vi "ObtainStopEvent.vi"() -> (3 "StopEvent":refnum<user-event>)   [LabVIEW 2014]
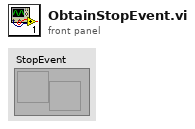
[diagram p1: front panel]
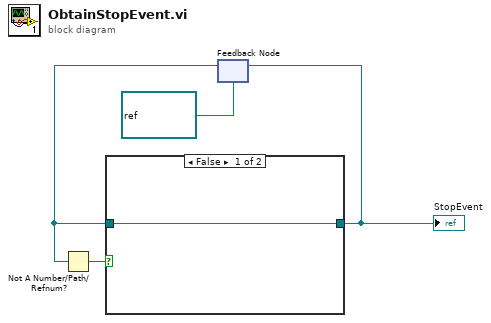
[diagram p0: block diagram]
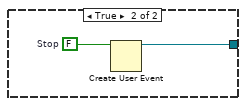
[diagram p2: hidden frame]
diagram:
  n1 = feedback #1(refnum<user-event> refnum ("Stop")) -> (w3:refnum<user-event>)
  n2 = Not A Number/Path/Refnum?(number/path/refnum=w3) -> (NaN/Path/Refnum?=w2:bool)
  n3 = case shown="False" w2 {
    tunnel: [w5 w6] -> w4
    tunnel: w3 -> [w5 _]
    frame False {
    }
    frame True {
      w7 = FALSE  # Stop
      n4 = Create User Event(user event datatype=w7) -> (user event=w6:refnum<user-event>)  [unwired: 1 in, 1 out]
    }
  }
  "StopEvent" <- w4
  n5 = feedback-in #1(w4) -> ()
